vi "Start Server.vi"(8 "error in (no error)":errorcluster, 11 "RemoteControl.STM in":refnum<class "RemoteControl.STM.lvclass">) -> (0 "error out":errorcluster, 3 "RemoteControl.STM out":refnum<class "RemoteControl.STM.lvclass">)   [LabVIEW 2016]
uses:
  ConnectionMonitor.vi
  RemoteControl.STM.lvclass
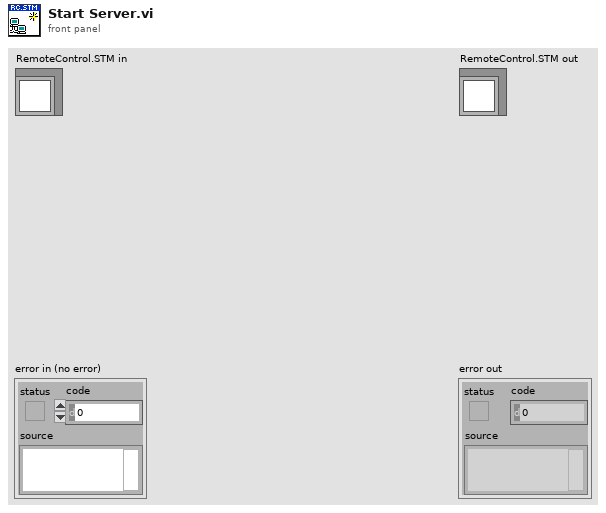
[diagram p1: front panel]
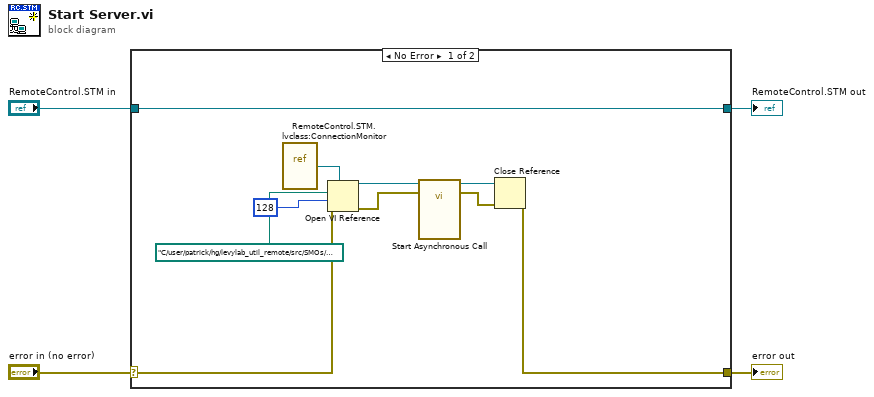
[diagram p0: block diagram]
diagram:
  n1 = case shown="No Error" "error in (no error)" {
    selector: "error in (no error)" -> [w10 w16]
    tunnel: [w5 w16] -> w3
    tunnel: [w14 w15] -> w1
    tunnel: "RemoteControl.STM in" -> [w14 w15]
    frame No Error {
      n2 = vi-ref "RemoteControl.STM.lvclass:ConnectionMonitor.vi"() -> (w12:refnum<vi>)
      n3 = Open VI Reference(type specifier VI Refnum (for type only)=w12, vi path=path "C:/user/patrick/hg/levylab_util_remote/src/SMOs/RemoteControl.STM/ConnectionMonitor.vi", options=128, error in (no error)=w10) -> (vi reference=w13:refnum<vi>, error out=w9:errorcluster)  [unwired: 2 in]
      n4 = call-by-ref "Start Asynchronous Call"(reference=w13, error in=w9) -> (reference out=w7:refnum<vi>, error out=w6:errorcluster)  [unwired: 12 in]
      n5 = Close Reference(reference=w7, error in (no error)=w6) -> (error out=w5:errorcluster)
    }
    frame Error {
    }
  }
  "error out" <- w3
  "RemoteControl.STM out" <- w1
